vi "Subarray Lorentz fit 2.vi"(6 "cursor diff":dbl, 9 "cursor avg":dbl, 10 "Y subset":dbl[](array[numeric]), 11 "X subset":dbl[](array[numeric])) -> (0 "error out":errorcluster, 1 "Initial params":dbl[](array[numeric]), 2 "best fit parameters":dbl[](array[numeric]), 3 "best nonlinear fit":dbl[](array[numeric]))   [LabVIEW 2015]
uses:
  <vilib>/gmath/NumericalOptimization/Nonlinear Curve Fit LM bound.vi
  <vilib>/gmath/NI_Gmath.lvlib
panel:
  # "Fitting to a more complicated Lorentzian-like function\n(called \"lfun3c\" in my Matlab functions):\nF = p(1)./((x-p(2)).^2+(p(3)^2)) + p(4)"
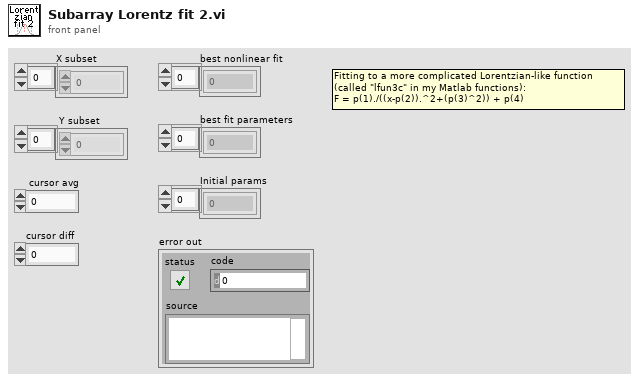
[diagram p1: front panel]
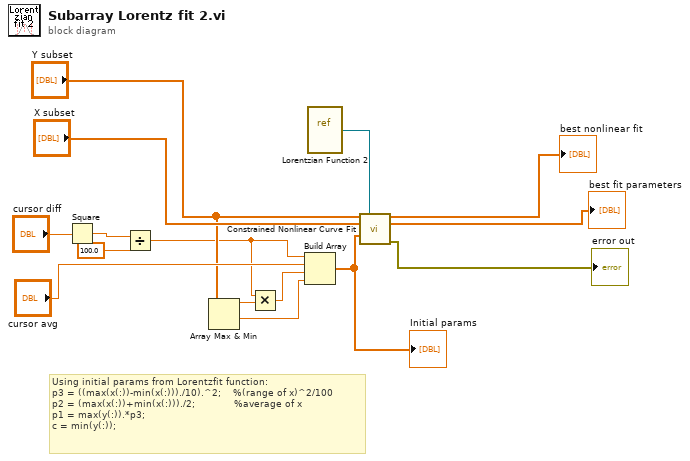
[diagram p0: block diagram]
diagram:
  # "Using initial params from Lorentzfit function:\np3 = ((max(x(:))-min(x(:)))./10).^2;    %(range of x)^2/100\np2 = (max(x(:))+min(x(:)))./2;             %average of x\np1 = max(y(:)).*p3;\nc = min(y(:));"
  n1 = Square(x="cursor diff") -> (x^2=w7:dbl)
  n2 = Divide(x=w7, y=100.0) -> (x/y=w2:dbl)
  n3 = Array Max & Min(array="Y subset") -> (max value=w4:dbl, min value=w3:dbl)  [unwired: 2 out]
  n4 = Multiply(x=w2, y=w4) -> (x*y=w1:dbl)
  n5 = Build Array(w2, "cursor avg", w1, w3) -> (w10:dbl[])
  "Initial params" <- w10
  n6 = vi-ref "Lorentzian Function 2.vi"() -> (w15:refnum<vi>)
  n7 = call-poly <vilib>:"Constrained Nonlinear Curve Fit.vi"("Y"="Y subset", "f(x,a)"=w15, "X"="X subset", "initial parameters"=w10) -> ("best nonlinear fit"=→"best nonlinear fit":dbl[], "best fit parameters"=→"best fit parameters":dbl[], "error out"=→"error out":errorcluster)  [unwired: 6 in, 3 out]
